vi "Legend Color.vi"(10 "label in":string, 11 "Flat Legend":cluster{"Color Box":u32, "String":string}[](array[cluster])) -> (2 "color out":u32)   [LabVIEW 2018]
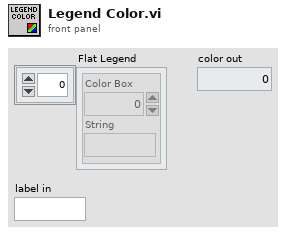
[diagram p1: front panel]
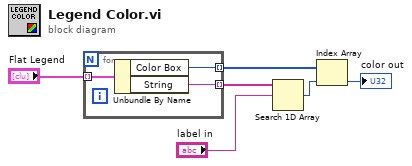
[diagram p0: block diagram]
diagram:
  n1 = for {
    tunnel: "Flat Legend" -> [w9] mode=indexing
    tunnel: [w8] -> w5 mode=indexing
    tunnel: [w7] -> w1 mode=indexing
    n2 = Unbundle By Name(w9) -> ("Color Box"=w8:u32, "String"=w7:string)
  }
  n3 = Search 1D Array(1D array=w1, element="label in") -> (index of element=w4:i32)  [unwired: 1 in]
  n4 = Index Array(array=w5, index=w4) -> (element=→"color out":u32)
